vi "Instrumentos Remotos.vi"() -> ()   [LabVIEW 2020]
uses:
  <vilib>/httpClient/LabVIEWHTTPClient.lvlib
panel:
  out "Lateral":bool
  out "Frontal":bool
  out "headers GET 2":string
  out "body GET 2":string
  in  "stop 2":bool
  out "error GET 2":errorcluster
  out "Temperatura":dbl
  out "Humedad":i32
  out "Fecha":string
  out "headers GET":string
  out "body GET":string
  in  "stop":bool
  out "error GET":errorcluster
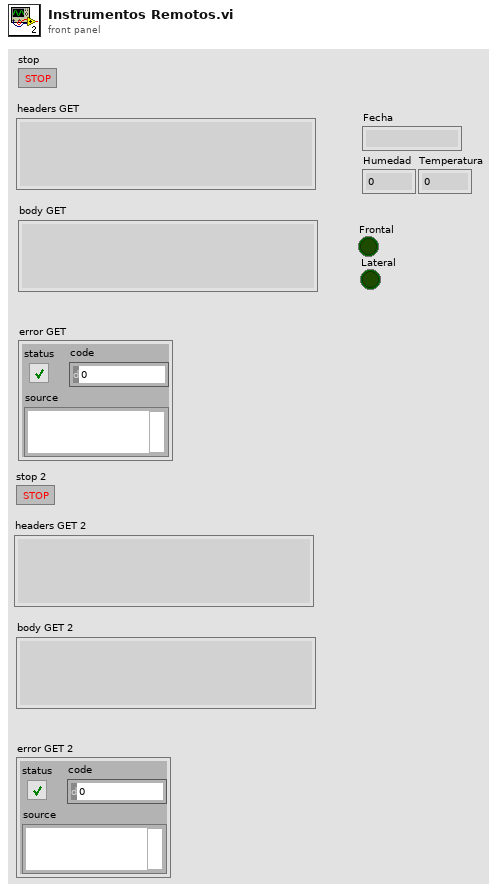
[diagram p1: front panel]
types:
  T1 = cluster{"Fecha":string, "Humedad":i32, "Temperatura":dbl}
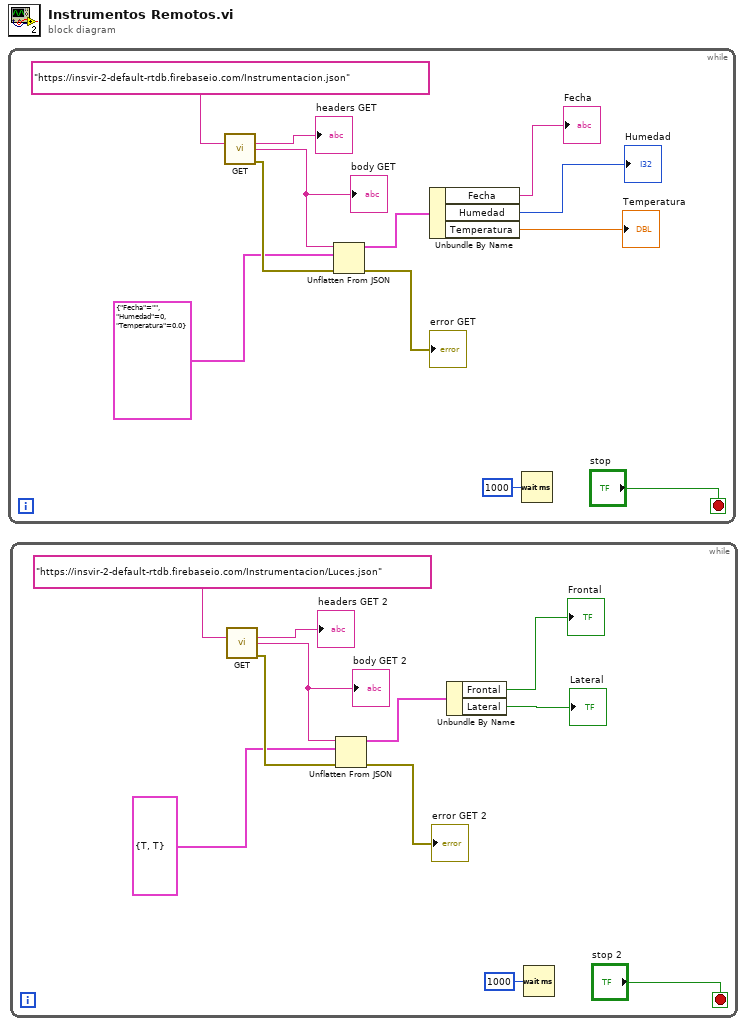
[diagram p0: block diagram]
diagram:
  n1 = while {
    stop <- "stop" stop-if-true
    n2 = call <vilib>:"GET.vi"("url"="https://insvir-2-default-rtdb.firebaseio.com/Instrumentacion.json") -> ("headers"=→"headers GET":string, "body"=w8:string, "error out"=w7:errorcluster)  [unwired: 11 in, 1 out]
    "body GET" <- w8
    n3 = Unflatten From JSON(JSON string=w8, type and defaults=T1 {"Fecha"="", "Humedad"=0, "Temperatura"=0.0}, error in (no error)=w7) -> (value=w4:T1, error out=→"error GET":errorcluster)  [unwired: 4 in]
    n4 = Unbundle By Name(w4) -> ("Fecha"=→"Fecha":string, "Humedad"=→"Humedad":i32, "Temperatura"=→"Temperatura":dbl)
    n5 = Wait (ms)(milliseconds to wait=u32 1000) -> ()  [unwired: 1 out]
  }
  n6 = while {
    stop <- "stop 2" stop-if-true
    n7 = call <vilib>:"GET.vi"("url"="https://insvir-2-default-rtdb.firebaseio.com/Instrumentacion/Luces.json") -> ("headers"=→"headers GET 2":string, "body"=w19:string, "error out"=w18:errorcluster)  [unwired: 11 in, 1 out]
    "body GET 2" <- w19
    n8 = Unflatten From JSON(JSON string=w19, type and defaults=cluster{"Frontal":bool, "Lateral":bool} {"Frontal"=TRUE, "Lateral"=TRUE}, error in (no error)=w18) -> (value=w15:cluster{"Frontal":bool, "Lateral":bool}, error out=→"error GET 2":errorcluster)  [unwired: 4 in]
    n9 = Unbundle By Name(w15) -> ("Frontal"=→"Frontal":bool, "Lateral"=→"Lateral":bool)
    n10 = Wait (ms)(milliseconds to wait=u32 1000) -> ()  [unwired: 1 out]
  }
